vi "Set Parameters.vi"(8 "Error In":errorcluster, 10 "Derived Parameters":T1 {"Phase Response [rad]" format="%#_4g"; "Amplitude Response" format="%#_4g"; "Angular Frequency [rad/s]" format="%#_4g"; "Time Constant [ms]" format="%#_4g"}, 11 "Derived Params Widget in":refnum<class "Derived Params Widget.lvclass">) -> (0 "Error Out":errorcluster, 3 "Derived Params Widget out":refnum<class "Derived Params Widget.lvclass">)   [LabVIEW 2014, in "Derived Params Widget.lvclass"]
doc: "Sets the parameters to be displayed.\n\n\nCopyright (c) 2019 Sze Howe Koh.\nThis code is licensed under the MIT license."
uses:
  Derived Params Widget.lvclass
  Derived Parameters.ctl
  Derived Params Widget.lvclass/Derived Params Widget.ctl
  <vilib>/addons/LQ/Qt Widgets/QDoubleSpinBox/QDoubleSpinBox.lvclass
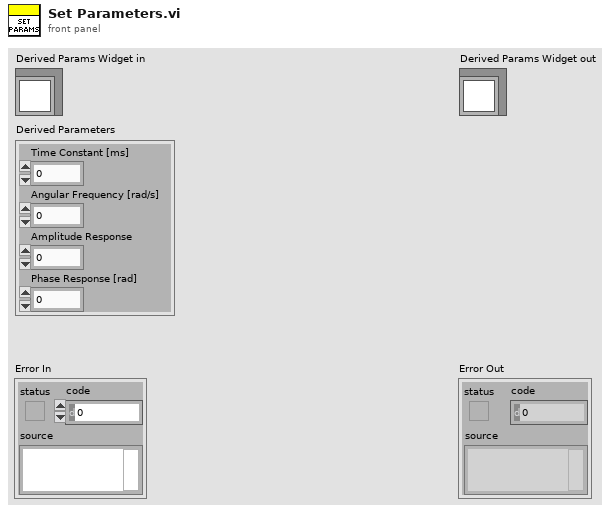
[diagram p1: front panel]
types:
  T1 = typedef "Derived Params Widget.lvclass/Derived Parameters.ctl" = cluster{"Time Constant [ms]":dbl, "Angular Frequency [rad/s]":dbl, "Amplitude Response":dbl, "Phase Response [rad]":dbl}
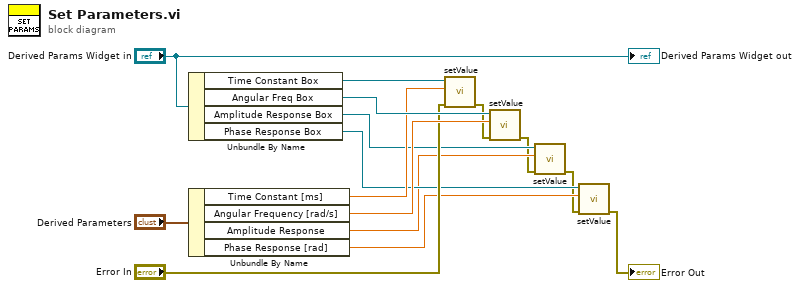
[diagram p0: block diagram]
diagram:
  n1 = Unbundle By Name("Derived Params Widget in") -> ("Time Constant Box"=w14:refnum<class "QDoubleSpinBox.lvclass">, "Angular Freq Box"=w13:refnum<class "QDoubleSpinBox.lvclass">, "Amplitude Response Box"=w7:refnum<class "QDoubleSpinBox.lvclass">, "Phase Response Box"=w6:refnum<class "QDoubleSpinBox.lvclass">)
  n2 = Unbundle By Name("Derived Parameters") -> ("Time Constant [ms]"=w11:dbl, "Angular Frequency [rad/s]"=w10:dbl, "Amplitude Response"=w5:dbl, "Phase Response [rad]"=w4:dbl)
  n3 = call <vilib>:"setValue.vi"("Error In"="Error In", "val"=w11, "QDoubleSpinBox In"=w14) -> ("Error Out"=w9:errorcluster)  [unwired: 7 in, 1 out]
  n4 = call <vilib>:"setValue.vi"("Error In"=w9, "val"=w10, "QDoubleSpinBox In"=w13) -> ("Error Out"=w3:errorcluster)  [unwired: 7 in, 1 out]
  n5 = call <vilib>:"setValue.vi"("Error In"=w3, "val"=w5, "QDoubleSpinBox In"=w7) -> ("Error Out"=w2:errorcluster)  [unwired: 7 in, 1 out]
  n6 = call <vilib>:"setValue.vi"("Error In"=w2, "val"=w4, "QDoubleSpinBox In"=w6) -> ("Error Out"=→"Error Out":errorcluster)  [unwired: 7 in, 1 out]
  "Derived Params Widget out" <- "Derived Params Widget in"
